vi "4 - Run lifecycle.vi"   [LabVIEW 2020]
uses:
  client/client.lvlib
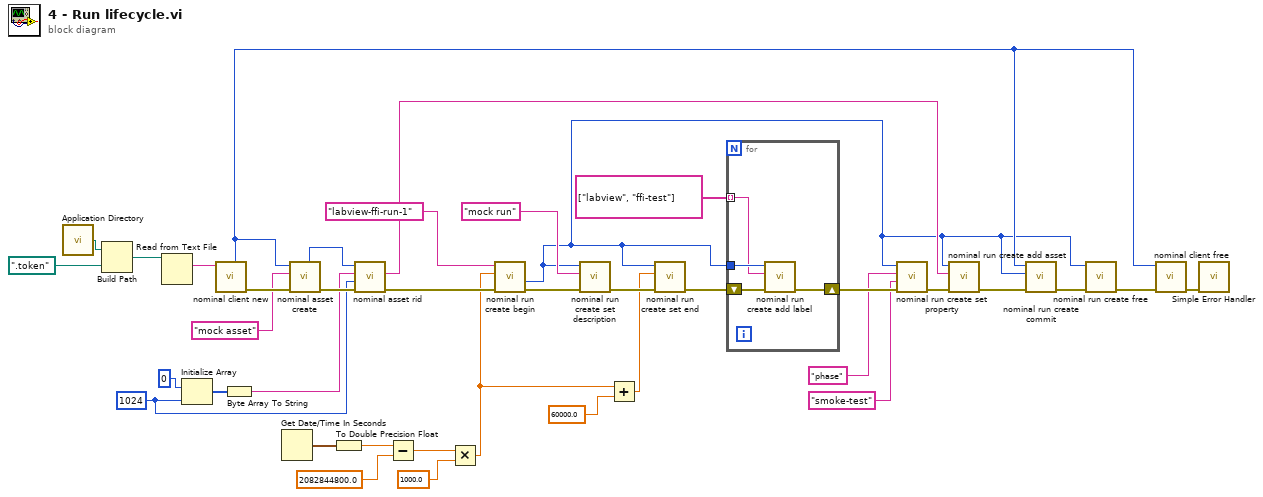
[diagram p0: block diagram]
diagram:
  w29 = 1024
  n1 = call <vilib>:"Application Directory.vi"() -> ("Application Directory"=w37:path)
  n2 = Build Path(base path=w37, name or relative path=path ".token") -> (appended path=w35:path)
  n3 = Read from Text File(file (use dialog)=w35) -> (text=w34:string)  [unwired: 3 in, 3 out]
  n4 = Initialize Array(u8 0, w29) -> (w28:u8[])
  n5 = call "nominal client new.vi"("token"=w34) -> ("error out"=w33:errorcluster, "out_client out"=w5:i32)  [unwired: 8 in, 1 out]
  n6 = Byte Array To String(unsigned byte array=w28) -> (string=w30:string)
  n7 = Get Date/Time In Seconds() -> (seconds since 1Jan1904=w21:timestamp)
  n8 = call "nominal asset create.vi"("error in (no error)"=w33, "name"="mock asset", "client"=w5) -> ("error out"=w31:errorcluster, "out_asset out"=w32:i32)  [unwired: 6 in, 1 out]
  n9 = To Double Precision Float(number=w21) -> (double precision float=w20:dbl)
  n10 = call "nominal asset rid.vi"("error in (no error)"=w31, "cap"=w29, "buf"=w30, "asset"=w32) -> ("error out"=w24:errorcluster, "buf out"=w7:string)  [unwired: 4 in, 2 out]
  n11 = Subtract(x=w20, y=2082844800.0) -> (x-y=w18:dbl)
  n12 = Multiply(x=w18, y=1000.0) -> (x*y=w15:dbl)
  n13 = call "nominal run create begin.vi"("error in (no error)"=w24, "start_ms"=w15, "name"="labview-ffi-run-1") -> ("error out"=w23:errorcluster, "out_staging out"=w3:i32)  [unwired: 6 in, 1 out]
  n14 = call "nominal run create set description.vi"("error in (no error)"=w23, "description"="mock run" ("name"), "staging"=w3) -> ("error out"=w16:errorcluster)  [unwired: 7 in, 1 out]
  n15 = Add(x=w15, y=60000.0) -> (x+y=w13:dbl)
  n16 = call "nominal run create set end.vi"("error in (no error)"=w16, "end_ms"=w13, "staging"=w3) -> ("error out"=w12:errorcluster)  [unwired: 7 in, 1 out]
  n17 = for {
    tunnel: w3 -> [w42]
    tunnel: string[] ["labview", "ffi-test"] ("name") -> [w40] mode=indexing
    shift-right: [w39] -> w10
    shift-left: w12 -> [w41]
    n18 = call "nominal run create add label.vi"("error in (no error)"=w41, "label"=w40, "staging"=w42) -> ("error out"=w39:errorcluster)  [unwired: 7 in, 1 out]
  }
  n19 = call "nominal run create set property.vi"("error in (no error)"=w10, "value"="smoke-test" ("name"), "key"="phase" ("name"), "staging"=w3) -> ("error out"=w6:errorcluster)  [unwired: 6 in, 1 out]
  n20 = call "nominal run create add asset.vi"("error in (no error)"=w6, "asset_rid"=w7, "staging"=w3) -> ("error out"=w4:errorcluster)  [unwired: 7 in, 1 out]
  n21 = call "nominal run create commit.vi"("error in (no error)"=w4, "staging"=w3, "client"=w5) -> ("error out"=w2:errorcluster)  [unwired: 6 in, 2 out]
  n22 = call "nominal run create free.vi"("error in (no error)"=w2, "staging"=w3) -> ("error out"=w1:errorcluster)  [unwired: 8 in, 1 out]
  n23 = call "nominal client free.vi"("error in (no error)"=w1, "client"=w5) -> ("error out"=w38:errorcluster)  [unwired: 8 in, 1 out]
  n24 = call <vilib>:"Simple Error Handler.vi"("error in (no error)"=w38) -> ()  [unwired: 4 in, 5 out]
